vi "Instrument Launch.vi"   [LabVIEW 2019]
uses:
  <vilib>/MGI/Panel Manager/Panel/Window Position/Reference Position/Alignment.ctl
  <vilib>/MGI/Panel Manager/Panel/Window Position/Reference Position/Horizontal Alignment.ctl
  <vilib>/MGI/Panel Manager/Panel/Window Position/Reference Position/Vertical Alignment.ctl
  Instrument/Instrument.lvclass
  C:/Program Files (x86)/National Instruments/LabVIEW 2019/vi.lib/MGI/Panel Manager/Panel Actor/Panel Actor/Panel Actor.lvclass
  Power Supply/Power Supply/Power Supply.lvclass
  C:/Working Copy/trunk/Modified Cobra Jung/Cobra/Cobra AF/Instrument/Instrument/Instrument.lvclass
  <vilib>/MGI/Panel Manager/Panel/Window Position/Reference Position/Offset/Absolute Offset/No Offset.vi
  <vilib>/MGI/Panel Manager/Panel/Window Position/Reference Position/Offset/Absolute Offset/Absolute Offset.lvclass
  C:/Program Files (x86)/National Instruments/LabVIEW 2019/vi.lib/MGI/Panel Manager/Panel/Window Position/Reference Position/Offset/Offset.lvclass
  <vilib>/MGI/Panel Manager/Panel/Window Position/Reference Position/Ref Display/Ref Display.lvclass
  C:/Program Files (x86)/National Instruments/LabVIEW 2019/vi.lib/MGI/Panel Manager/Panel/Window Position/Window Position.lvclass
  <vilib>/MGI/Panel Manager/Panel/Window Position/Reference Position/Ref Display/Ref Display.vi
  <vilib>/MGI/Panel Manager/Panel Actor/Panel Actor/Launch Root Panel Window.vi
  <vilib>/MGI/Panel Manager/Panel Actor/Panel Actor/Panel Actor.lvclass
  <vilib>/MGI/Panel Manager/Panel/Panel.lvlib
  <vilib>/MGI/Panel Manager/Panel/Window Position/Reference Position/Reference Position.lvclass
  C:/Program Files (x86)/National Instruments/LabVIEW 2019/vi.lib/MGI/Panel Manager/Panel/Window Position/Reference Position/Reference Position.lvclass
  C:/Program Files (x86)/National Instruments/LabVIEW 2019/vi.lib/MGI/Monitored Actor/Monitored Actor/Monitored Actor/Monitored Actor.lvclass
  C:/Program Files (x86)/National Instruments/LabVIEW 2019/vi.lib/ActorFramework/Actor/Actor.lvclass
panel:
  # "Instrument Testing"
types:
  T1 = typedef "Panel.lvlib/Reference Position.lvclass/Alignment.ctl" = cluster{"Horizontal":T2, "Vertical":T3}
  T2 = typedef "Panel.lvlib/Reference Position.lvclass/Horizontal Alignment.ctl" = enum16{"Left", "Center", "Right"}
  T3 = typedef "Panel.lvlib/Reference Position.lvclass/Vertical Alignment.ctl" = enum16{"Top", "Center", "Bottom"}
  T4 = enum32{"Invalid", "Standard", "Closed", "Hidden", "Minimized", "Maximized"}
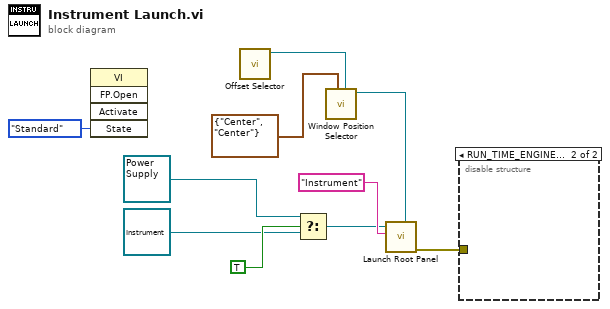
[diagram p0: block diagram]
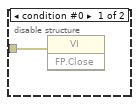
[diagram p2: hidden frame]
diagram:
  n1 = invoke class="VI" method="FP.Open"("State"=T4."Standard") -> ()  [unwired: 4 in, 5 out]
  n2 = call-poly <vilib>:"Offset Selector.vi"() -> ("Absolute Offset Out"=w4:refnum<class "Absolute Offset.lvclass">)  [unwired: 10 in, 1 out]
  n3 = Select(t=refnum<class "Power Supply.lvclass"> refnum ("Power Supply.lvlib:Power Supply.lvclass"), s=TRUE, f=refnum<class "Instrument.lvclass"> refnum ("Instrument.lvlib:Instrument.lvclass")) -> (s? t:f=w6:refnum<class "Instrument.lvclass">)
  n4 = call-poly <vilib>:"Window Position Selector.vi"("Offset"=w4, "Alignment"=T1 {"Horizontal"=enum."Center", "Vertical"=enum."Center"}) -> ("Ref Display out"=w9:refnum<class "Ref Display.lvclass">)  [unwired: 8 in, 1 out]
  n5 = call-poly <vilib>:"Launch Root Panel.vi"("Window Position (Maximize First Call)"=w9, "Title"="Instrument", "Panel Actor in"=w6) -> ("Error Out"=w10:errorcluster)  [unwired: 7 in, 1 out]
  n6 = disable-structure shown="RUN_TIME_ENGINE==False" {
    disable-tunnel: w10 -> [w11 _]
    frame condition #0 {
      n7 = invoke class="VI" method="FP.Close"(error in=w11) -> ()  [unwired: 2 in, 3 out]
    }
    frame condition #1 (active) {
    }
  }
